vi "marshalling.vi"(8 "error in (no error)":errorcluster, 10 "Variant":variant, 11 "Serializer in":refnum<class "Serializer.Template.lvclass">) -> (0 "error out":errorcluster, 2 "String":string, 3 "Serializer":refnum<class "Serializer.Template.lvclass">)   [LabVIEW 2013, in "OpenSerializer.Template.lvlib" / "Serializer.Template.lvclass"]
uses:
  Serializer.Template.lvclass
  <vilib>/LabVIEW Open Source Project/OpenSerializer/Serializer/Serializer.lvclass
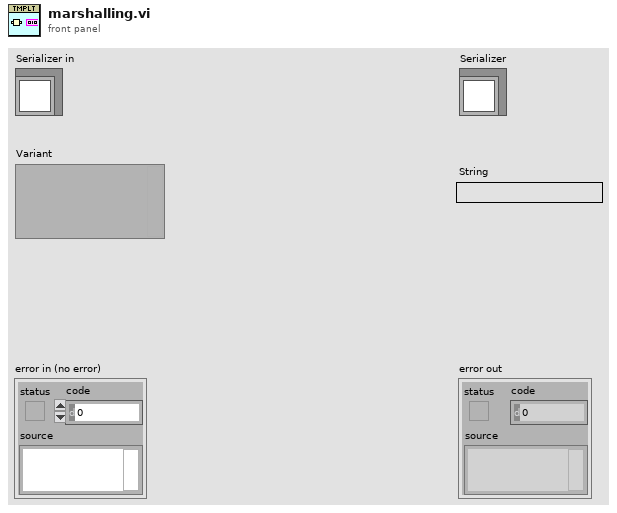
[diagram p1: front panel]
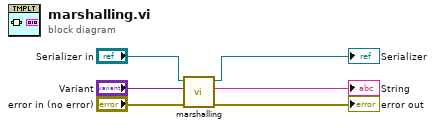
[diagram p0: block diagram]
diagram:
  n1 = call-parent "marshalling.vi"("error in (no error)"="error in (no error)", "Variant"="Variant", "Serializer in"="Serializer in") -> ("error out"=→"error out":errorcluster, "String"=→"String":string, "Serializer out"=→"Serializer":refnum<class "Serializer.Template.lvclass">)  [unwired: 6 in]
